vi "DFD Filter Array.vi"(7 "init (F)":bool, 8 "error in (no error)":errorcluster, 10 "IIR Filters":T1(array[cluster]), 11 "signal in":waveform(dbl)[](array[waveform])) -> (0 "error out":errorcluster, 3 "signal out":waveform(dbl)[](array[waveform]))   [LabVIEW 2019, in "DSP.lvclass"]
uses:
  DSP.lvclass
  Typedefs/Filter State--Cluster.ctl
  <vilib>/Analysis/3filter.llb/IIR Cascade Filter with I.C. (DBL).vi
  <vilib>/Analysis/NI_AALBase.lvlib
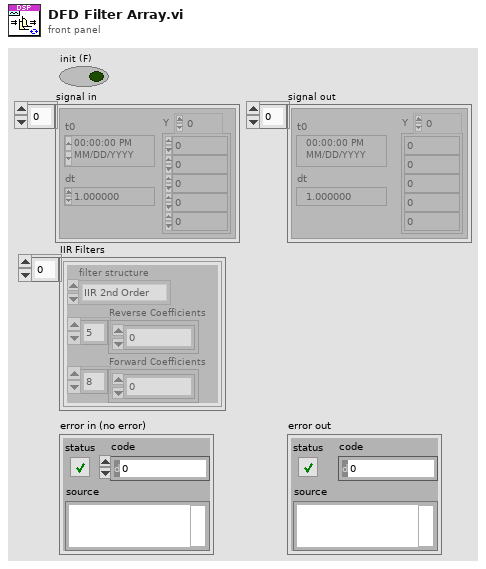
[diagram p1: front panel]
types:
  T1 = cluster{"filter structure":enum32{"IIR 2nd Order", "IIR 4th Order"}, "Reverse Coefficients":dbl[], "Forward Coefficients":dbl[]}[]
  T2 = typedef "DSP.lvclass/Filter State--Cluster.ctl" = cluster{"Filter State":dbl[]}
  T3 = cluster{"filter structure":enum32{"IIR 2nd Order", "IIR 4th Order"}, "Reverse Coefficients":dbl[], "Forward Coefficients":dbl[]}
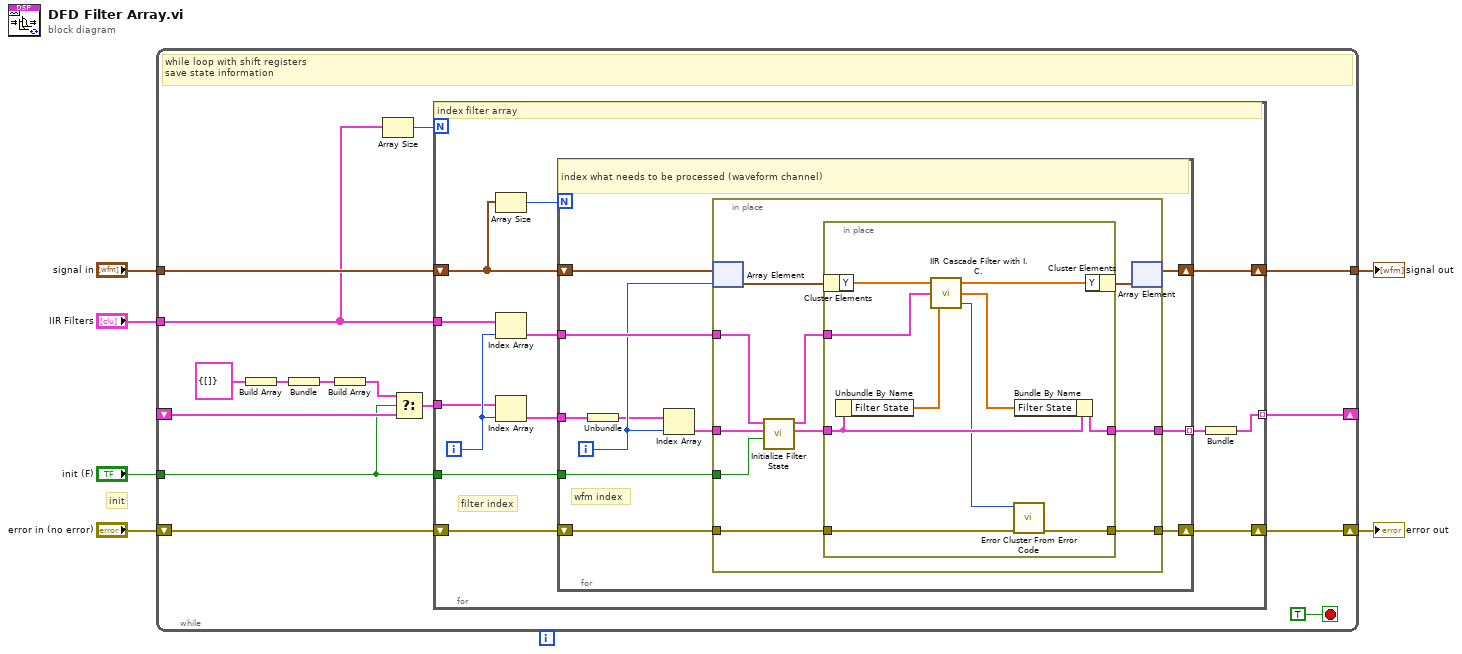
[diagram p0: block diagram]
diagram:
  # "init"
  n1 = while {
    tunnel: "init (F)" -> [w7]
    tunnel: "IIR Filters" -> [w10]
    tunnel: "signal in" -> [w17]
    tunnel: [w21] -> w2
    shift-right: [w20] -> w3
    shift-left: "error in (no error)" -> [w18]
    shift-right: [w8] -> _
    shift-left: _ -> [w9]
    stop <- TRUE stop-if-true
    # "while loop with shift registers \nsave state information"
    n2 = Build Array(T2 {"Filter State"=[]} ("s? t:f")) -> (w13:T2[])
    n3 = Bundle(w13) -> (w14:cluster{T2[]})  [unwired: 1 in]
    n4 = Build Array(w14) -> (w12:cluster{T2[]}[])
    n5 = Array Size(array=w10) -> (size(s)=w11:i32)
    n6 = Select(t=w12, s=w7, f=w9) -> (s? t:f=w15:cluster{T2[]}[])
    n7 = for {
      N: w11 -> [_]
      tunnel: w10 -> [w30]
      tunnel: w7 -> [w27]
      tunnel: [w22] -> w8 mode=indexing
      tunnel: w15 -> [w24]
      shift-right: [w33] -> w20
      shift-left: w18 -> [w32]
      shift-right: [w34] -> w21
      shift-left: w17 -> [w31]
      i -> [w26]
      # "filter index"
      # "index filter array"
      n8 = Array Size(array=w31) -> (size(s)=w29:i32)
      n9 = Index Array(array=w30, index=w26) -> (element=w28:T3)
      n10 = Index Array(array=w24, index=w26) -> (element=w25:cluster{T2[]})
      n11 = for {
        N: w29 -> [_]
        shift-right: [w44] -> w33
        shift-left: w32 -> [w45]
        shift-right: [w42] -> w34
        shift-left: w31 -> [w43]
        tunnel: w27 -> [w41]
        tunnel: w28 -> [w40]
        tunnel: [w39] -> w23 mode=indexing
        tunnel: w25 -> [w36]
        i -> [w38]
        # "wfm index"
        # "index what needs to be processed (waveform channel)"
        n12 = Unbundle(w36) -> (w35:T2[])
        n13 = Index Array(array=w35, index=w38) -> (element=w37:T2)
        n14 = in-place {
          in-place-border: w45 -> [w55]
          in-place-border: [w54] -> w44
          in-place-border: w41 -> [w51]
          in-place-border: w40 -> [w48]
          in-place-border: [w47] -> w39
          in-place-border: w37 -> [w46]
          n15 = in-place-array #1(w43, w38) -> (w53:waveform(dbl))
          n16 = call "Initialize Filter State.vi"("init (F)"=w51, "Filter State in"=w46, "IIR Filter Cluster"=w48) -> ("Filter State out"=w50:T2, "IIR Filter Cluster"=w49:T3)  [unwired: 7 in]
          n17 = in-place {
            in-place-border: w55 -> [w65]
            in-place-border: [w64] -> w54
            in-place-border: [w60] -> w47
            in-place-border: w50 -> [w61]
            in-place-border: w49 -> [w57]
            n18 = in-place-cluster #2(w53) -> ("Y"=w63:dbl[])
            n19 = Unbundle By Name(w61) -> ("Filter State"=w62:dbl[])
            n20 = call-poly <vilib>:"IIR Cascade Filter with I.C..vi"("Initial Filter State"=w62, "IIR Filter Cluster"=w57, "X"=w63) -> ("error"=w56:i32, "Final Filter State"=w58:dbl[], "Filtered X"=w59:dbl[])
            n21 = call <vilib>:"Error Cluster From Error Code.vi"("error in (no error)"=w65, "error code (0)"=w56) -> ("error out"=w64:errorcluster)  [unwired: 7 in]
            n22 = Bundle By Name(cluster=w61, "Filter State"=w58) -> (w60:T2)
            n23 = in-place-cluster #2("Y"=w59) -> (w52:waveform(dbl))
          }
          n24 = in-place-array #1(w52) -> (w42:waveform(dbl)[])  [unwired: 1 out]
        }
      }
      n25 = Bundle(w23) -> (w22:cluster{T2[]})  [unwired: 1 in]
    }
  }
  "error out" <- w3
  "signal out" <- w2
